vi "Tosca-Remap Schedule Variables.vi"(0 "Schedule in":T1, 11 "error in (no error)":errorcluster, 12 "AO Name Map":cluster{"old":string[], "new":string[]}) -> (4 "Schedule out":T1, 15 "error out":errorcluster)   [LabVIEW 2015]
uses:
  Typedefs/Tosca-Schedule.ctl
  Typedefs/Tosca-Sequence Order.ctl
  Typedefs/Tosca-Parameter Family.ctl
  Typedefs/Tosca-Parameter Table Element.ctl
  Typedefs/Tosca-Parameter Dimension.ctl
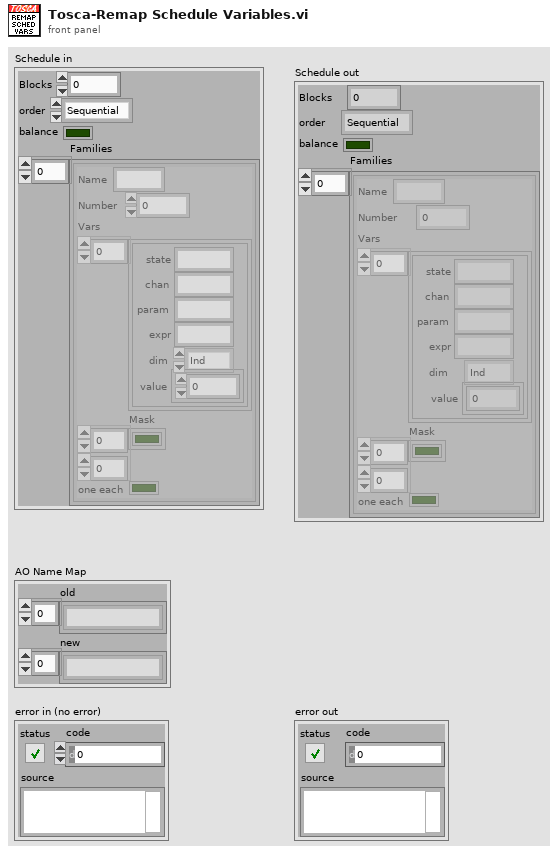
[diagram p1: front panel]
types:
  T1 = typedef "Tosca-Schedule.ctl" = cluster{"Blocks":i32, "order":T2, "balance":bool, "Families":T3[]}
  T2 = typedef "Tosca-Sequence Order.ctl" = enum16{"Sequential", "Alternate", "Randomize", "Random group"}
  T3 = typedef "Tosca-Parameter Family.ctl" = cluster{"Name":string, "Number":i32, "Vars":T4[], "Mask":bool[][], "one each":bool}
  T4 = typedef "Tosca-Parameter Table Element.ctl" = cluster{"state":string, "chan":string, "param":string, "expr":string, "dim":T5, "value":dbl[]}
  T5 = typedef "Tosca-Parameter Dimension.ctl" = enum16{"Ind", "X", "Y"}
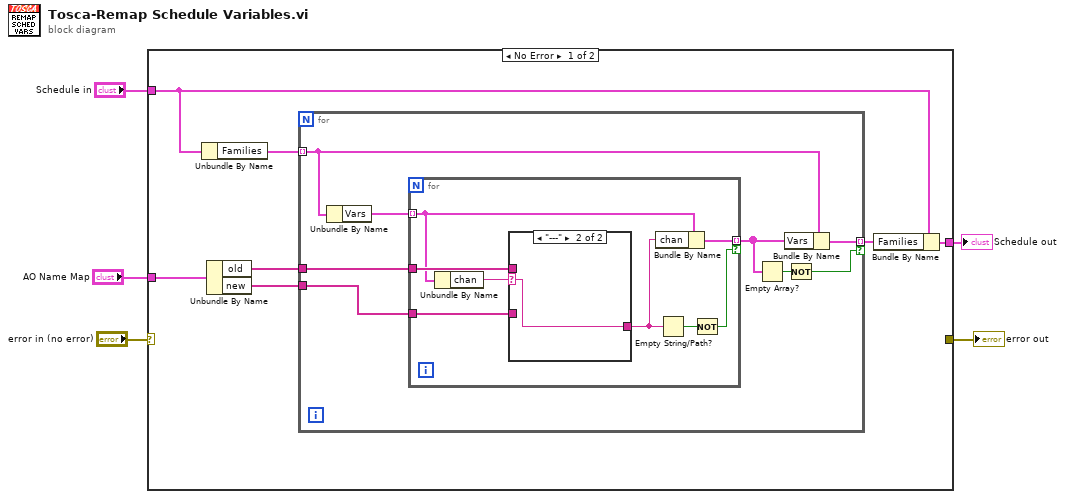
[diagram p0: block diagram]
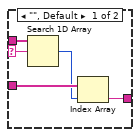
[diagram p2: hidden frame]
diagram:
  n1 = case shown="No Error" "error in (no error)" {
    selector: "error in (no error)" -> [_ w35]
    tunnel: "AO Name Map" -> [w12 _]
    tunnel: "Schedule in" -> [w8 w36]
    tunnel: [w6 w36] -> w3
    tunnel: [_ w35] -> w1
    frame No Error {
      n2 = Unbundle By Name(w8) -> ("Families"=w11:T3[])
      n3 = Unbundle By Name(w12) -> ("old"=w10:string[], "new"=w9:string[])
      n4 = for {
        tunnel: w11 -> [w17] mode=indexing
        tunnel: w10 -> [w20]
        tunnel: w9 -> [w19]
        tunnel: [w16] -> w7 mode=indexing if=w13
        n5 = Unbundle By Name(w17) -> ("Vars"=w18:T4[])
        n6 = for {
          tunnel: w18 -> [w26] mode=indexing
          tunnel: w20 -> [w28]
          tunnel: w19 -> [w27]
          tunnel: [w25] -> w15 mode=indexing if=w22
          n7 = Unbundle By Name(w26) -> ("chan"=w21:string)
          n8 = case shown="\"---\"" w21 {
            selector: w21 -> [w29 w34]
            tunnel: w28 -> [w33 _]
            tunnel: w27 -> [w32 _]
            tunnel: [w30 w34] -> w24
            frame "", Default {
              n9 = Search 1D Array(1D array=w33, element=w29) -> (index of element=w31:i32)  [unwired: 1 in]
              n10 = Index Array(array=w32, index=w31) -> (element=w30:string)
            }
            frame "---" {
            }
          }
          n11 = Bundle By Name(cluster=w26, "chan"=w24) -> (w25:T4)
          n12 = Empty String/Path?(string/path=w24) -> (empty?=w23:bool)
          n13 = Not(x=w23) -> (.not. x?=w22:bool)
        }
        n14 = Empty Array?(array=w15) -> (empty?=w14:bool)
        n15 = Bundle By Name(cluster=w17, "Vars"=w15) -> (w16:T3)
        n16 = Not(x=w14) -> (.not. x?=w13:bool)
      }
      n17 = Bundle By Name(cluster=w8, "Families"=w7) -> (w6:T1)
    }
    frame Error {
    }
  }
  "Schedule out" <- w3
  "error out" <- w1
